vi "Error Query (multiple).vi"(8 "error in (no error)":errorcluster, 11 "VISA resource name":refnum<visa-resource-name>) -> (0 "error out":errorcluster, 1 "error message":string, 2 "error":bool, 3 "VISA resource name out":refnum<visa-resource-name>)   [LabVIEW 2012, in "Agilent E364X Series.lvlib"]
doc: "This VI reads the error queue from the instrument. It expects to see errors in SCPI format (#,\"error message\"). It continues to read from the error queue until it reads a 0, \"No error\"."
uses:
  Agilent E364X Series.lvlib
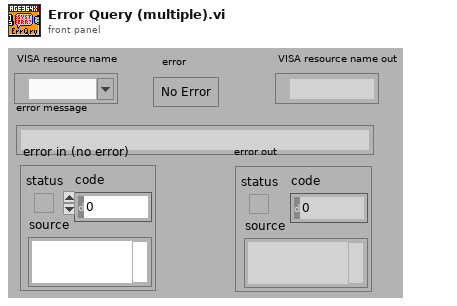
[diagram p1: front panel]
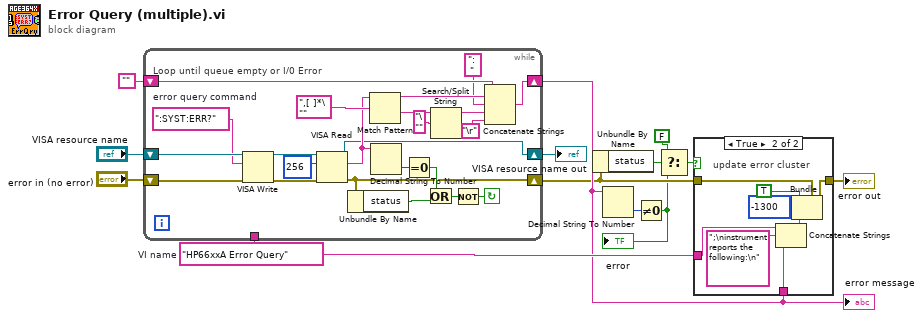
[diagram p0: block diagram]
diagram:
  w12 = "HP66xxA Error Query"  # VI name
  n1 = while {
    shift-left: "VISA resource name" -> [w33]
    shift-right: [w19] -> w11
    tunnel: w12 -> [_]
    shift-left: "error in (no error)" -> [w34]
    shift-right: [w20] -> w5
    shift-left: "" -> [w36]
    shift-right: [w18] -> w9
    stop <- w35 continue-if-true
    w28 = ":SYST:ERR?"  # error query command
    # "Loop until queue empty or I/0 Error"
    n2 = VISA Write(VISA resource name=w33, write buffer=w28, error in (no error)=w34) -> (VISA resource name out=w27:refnum<visa-resource-name>, error out=w26:errorcluster)  [unwired: 1 out]
    n3 = VISA Read(VISA resource name=w27, byte count=u32 256, error in (no error)=w26) -> (VISA resource name out=w19:refnum<visa-resource-name>, read buffer=w21:string, error out=w20:errorcluster)  [unwired: 1 out]
    n4 = Unbundle By Name(w20) -> ("status"=w30:bool)
    n5 = Match Pattern(string=w21, regular expression=",[ ]*\"") -> (before substring=w24:string, after substring=w22:string)  [unwired: 1 in, 2 out]
    n6 = Decimal String To Number(string=w21) -> (number=w32:i32)  [unwired: 2 in, 1 out]
    n7 = Equal To 0?(x=w32) -> (x = 0?=w31:bool)
    n8 = Or(x=w31, y=w30) -> (x .or. y?=w17:bool)
    n9 = Search/Split String(string=w22, search string/char (-)="\"") -> (substring before match=w15:string)  [unwired: 1 in, 2 out]
    n10 = Not(x=w17) -> (.not. x?=w35:bool)
    n11 = Concatenate Strings(w36, w24, ":  ", w15, "\r") -> (w18:string)
  }
  "error message" <- w9
  "VISA resource name out" <- w11
  n12 = Unbundle By Name(w5) -> ("status"=w3:bool)
  n13 = Decimal String To Number(string=w9) -> (number=w10:i32)  [unwired: 2 in, 1 out]
  n14 = Not Equal To 0?(x=w10) -> (x != 0?=w2:bool)
  "error" <- w2
  n15 = Select(t=FALSE, s=w3, f=w2) -> (s? t:f=w1:bool)
  n16 = case shown="True" w1 {
    tunnel: w5 -> [w37 w43]
    tunnel: [w37 w42] -> w8
    tunnel: w9 -> [_ w39]
    tunnel: w12 -> [_ w38]
    frame False {
      # "no instrument errors"
    }
    frame True {
      # "update error cluster"
      n17 = Concatenate Strings(w38, ";\ninstrument reports the following:\n", w39) -> (w41:string)
      n18 = Bundle(cluster=w43, "status"=TRUE, "code"=-1300, "source"=w41) -> (w42:errorcluster)
    }
  }
  "error out" <- w8
